vi "2_1_Face_Detection_Eval(CPU,GPU).vi"() -> ()   [LabVIEW 2020]
doc: "This example demonstrates the usage of the \"DeepLTK FPGA Addon\" for deploying a Face Detection model on a PXI-FPGA board, utilizing an input image sourced from a file.\n\nMore Examples: https://github.com/ngenehub/deepltk_fpga_examples"
uses:
  <vilib>/Ngene/Deep Learning Toolkit/Toolkit/NN_Network/Controls/NN_Device.ctl
  <vilib>/Ngene/Deep Learning Toolkit/Toolkit/NN_Network/Controls/NN_Save_Before_Destroy_Options.ctl
  723d4076-311b-47b4-ac66-0871b538cff2.vi
  <vilib>/Ngene/Deep Learning Toolkit/Toolkit/NN_Data/subVIs/Dataset/NN_Variant_to_DVR/4D/NN_Data_Variant_to_DVR(4D_SGL).vi
  <vilib>/Ngene/Deep Learning Toolkit/Toolkit/NN_Data/subVIs/Get_Data_Vals/4D/NN_Data_Get_ValByRef(4D_SGL_idx).vi
  <vilib>/Ngene/Deep Learning Toolkit/Toolkit/NN_Network/API/NN_Set_Input/3D/NN_Set_Input(3D_SGL_idx).vi
  <vilib>/Ngene/Deep Learning Toolkit/Toolkit/NN_Train/Eval_Loss/NN_Eval_Test_Error_Loss/NN_Eval(In3D_OutBBox).vi
  <vilib>/Ngene/Deep Learning Toolkit/Toolkit/NN_Train/Eval_Loss/NN_Calc_Cofusion_Matrix/NN_Calc_Confusion_Matrix(In3D_OutBBox).vi
  <vilib>/Ngene/Deep Learning Toolkit/Toolkit/Deep_Learning_Toolkit_by_Ngene.lvlib
  <vilib>/ptbypt/NI_PtbyPt.lvlib
panel:
  out "Eval Time":dbl=0.10011647000010271 format="%#_2p"
  out "Loop time":dbl=0.10057269999997516 format="%#_2p"
  out "Confusion Matrix":string[][](table)=[["24", "10", "0.7059"], ["8", "0", "0.0000"], ["0.7500", "0.0000", ""]]
  out "Iterations":i32=13
  out "Dataset Size":i32=14
  in  "NN_Device":T1
  in  "Stop":bool
  in  "Dataset Path (Annotations)":path=path "D:/Ngene/GitHub/deepltk_fpga_examples/2_Face_Detection(PXI,sbRIO)/Dataset/Annotations"
  out "mAP@0.5":sgl=0.72716737
  out "mIOU":sgl=0.5610681
  in  "Display?":bool
  out "Display":T2(plugin-control)
  in  "Dataset Path (Images)":path=path "D:/Ngene/GitHub/deepltk_fpga_examples/2_Face_Detection(PXI,sbRIO)/Dataset/Images"
  in  "Confidence_Thresh":sgl=0.46
  in  "IOU_Thresh":sgl=0.4
  in  "Weight File Path":path=path "D:/Ngene/GitHub/deepltk_fpga_examples/2_Face_Detection(PXI,sbRIO)/Models/Face_Detection_Original/Face_Detection.bin"
  in  "Configuration File Path":path=path "D:/Ngene/GitHub/deepltk_fpga_examples/2_Face_Detection(PXI,sbRIO)/Models/Face_Detection_Original/Face_Detection.cfg"
  # "Overview: This VI is designed to evaluate (measure the accuracy of) a pretrained object detection model.\nRequirements: \n• DeepLTK - Deep Learning Toolkit for LabVIEW (https://www.ngene.co/deep-learning-toolkit-for-labview)\n• NI Vision Development Module\nInstructions:\n1.\tProvide the path to the dataset to be evaluated at Dataset. A sample is available in the \"Dataset\" folder. \n2.\tProvide the \"Network Configuration File Path\" and \"Weight File Path\" locted in \"Models\\Face_Detection_Original\" folder in the project.\n3. Use NN_Device to specify the device (CPU or GPU) for execution. GPU is applicable only for 64-bit LabVIEW.\n4.\tRun the VI.\n5.\tObserve measured accuracy at mIOU, mAP@0.5 and Confusion Matrix indicators."
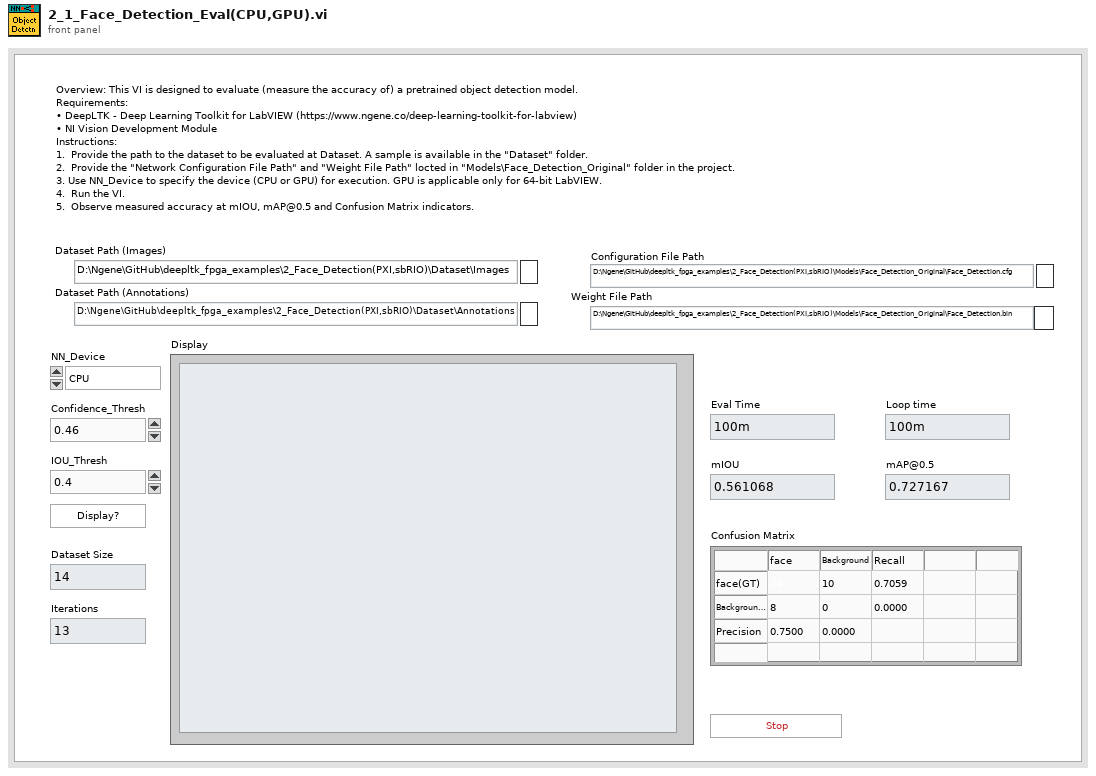
[diagram p1: front panel]
types:
  T1 = typedef "Deep_Learning_Toolkit_by_Ngene.lvlib/NN_Device.ctl" = enum16{"CPU", "GPU"}
  T2 = typedef "IMAQ Image.ctl" = refnum<image>
  T3 = typedef "Deep_Learning_Toolkit_by_Ngene.lvlib/NN_Save_Before_Destroy_Options.ctl" = cluster{"CFG?":bool, "Weights?":bool, "Render?":bool}
  T4 = typedef "Image Type" = u32
  T5 = typedef "Deep_Learning_Toolkit_by_Ngene.lvlib/NN_Config_Params.ctl" = cluster{"Name":string, "mBatch":i32, "NN_Train_Params":T6, "LR_Decay_Policy":T9, "Labels":string[], "Loss":T11}
  T6 = typedef "Deep_Learning_Toolkit_by_Ngene.lvlib/NN_Train_Params.ctl" = cluster{"Optimizer":T7, "Beta_1":sgl, "Beta_2":sgl, "Weight Decay(L1)":sgl, "Weight Decay(L2)":sgl, "Data_Sampling":T8}
  T7 = typedef "Deep_Learning_Toolkit_by_Ngene.lvlib/NN_Train_Optimizer.ctl" = enum16{"SGD", "Adam", "Adagrad", "Adadelta", "RMSProp", "Nesterov"}
  T8 = typedef "Deep_Learning_Toolkit_by_Ngene.lvlib/NN_Train_Data_Sampling.ctl" = enum16{"Random", "Sequential"}
  T9 = typedef "Deep_Learning_Toolkit_by_Ngene.lvlib/NN_LR_Policy_Cfg.ctl" = cluster{"Policy_Type":T10, "LR0":dbl, "k":sgl, "WarmUp_Policy":enum16{"Step", "Ramp"}, "WarmUp_Iter":i32, "WarmUp_Ratio":sgl}
  T10 = typedef "Deep_Learning_Toolkit_by_Ngene.lvlib/NN_LR_Policy_Type.ctl" = enum16{"Manual", "Step", "Exp", "1/t"}
  T11 = typedef "Deep_Learning_Toolkit_by_Ngene.lvlib/NN_Loss_Config_Params.ctl" = cluster{"Loss_Type":T12, "Loss_Conf_Params":variant}
  T12 = typedef "Deep_Learning_Toolkit_by_Ngene.lvlib/NN_Loss_Type.ctl" = enum16{"None", "MSE", "CrossEntropy", "YOLO_v2", "YOLO_v4"}
  T13 = typedef "Deep_Learning_Toolkit_by_Ngene.lvlib/NN_Layer_Config_Params.ctl" = cluster{"Layer_Type":T14, "Layer_Conf_Params":variant, "Input Layers":string[]}
  T14 = typedef "Deep_Learning_Toolkit_by_Ngene.lvlib/NN_Layer_Type.ctl" = enum16{"Input1D", "Input3D", "Conv1D", "Conv2D", "Conv2D_Adv", "MaxPool", "AvgPool", "UpSample", "DropOut3D", "ShortCut", "Concat", "SoftMax3D", "FC", "DropOut", "Softmax", "Flatten", "YOLO_v2", "YOLO_v4", "Activation", "BatchNormalization", "Unsupported"}
  T15 = typedef "Deep_Learning_Toolkit_by_Ngene.lvlib/NN.ctl" = cluster{"Name":string, "No of Layers":i32, "mBatch":i32, "Layers":T16[], "Dimty":T17, "Dims_In":T18, "Dims_Out":T18, "Working_Dir":path, "Train?":bool, "Train_Params":T6, "LR_Update_Policy":T9, "Session Data":T19, "Ground_truth":T20, "NNg_hdls":T21, "NN_Device":T1, "GPU Id":i32, "Labels":string[], "Receptive Field":T22[], "Loss_Type":T12, "Loss_Cfg_Prms":variant, "NNG_WS":T23}
  T16 = typedef "Deep_Learning_Toolkit_by_Ngene.lvlib/NN_Layer_ref.ctl" = refnum<data-value>
  T17 = typedef "Deep_Learning_Toolkit_by_Ngene.lvlib/NN_In_Out_Dim-ty.ctl" = enum8{"In1D_Out1D", "In3D_Out1D", "In3D_Out3D", "In3D_OutBBox"}
  T18 = typedef "Deep_Learning_Toolkit_by_Ngene.lvlib/NN_Dims(C,H,W).ctl" = cluster{"C":i32, "H":i32, "W":i32}
  T19 = typedef "Deep_Learning_Toolkit_by_Ngene.lvlib/NN_Train_Session_Data.ctl" = cluster{"Epochs":sgl, "Tot_Iter":i32, "LR":sgl, "LR_iter":i32}
  T20 = typedef "Deep_Learning_Toolkit_by_Ngene.lvlib/NN_Ground_truth.ctl" = cluster{"Y":variant}
  T21 = typedef "Deep_Learning_Toolkit_by_Ngene.lvlib/nng_cuda_handles.ctl" = cluster{"cudnn":u64, "cublas":u64, "stream":u64, "curand":u64}
  T22 = typedef "Deep_Learning_Toolkit_by_Ngene.lvlib/NN_Dims(V,H).ctl" = cluster{"V":i32, "H":i32}
  T23 = typedef "Deep_Learning_Toolkit_by_Ngene.lvlib/NNG_WS.ctl" = cluster{"NNG_WS_Mem":T24, "Max_WS_Size":i64}
  T24 = typedef "Deep_Learning_Toolkit_by_Ngene.lvlib/NNg_WS_Mem_DVR.ctl" = refnum<data-value>
  T25 = typedef "Deep_Learning_Toolkit_by_Ngene.lvlib/NN_DataSets_All(In3D_OutBBox).ctl" = cluster{"Train":T26, "Validation":T26, "Test":T26}
  T26 = typedef "Deep_Learning_Toolkit_by_Ngene.lvlib/NN_DataSet(In3D_OutBBox).ctl" = cluster{"Inputs Ref.":variant, "Dataset_Size":i32, "Dims_In":T18, "Outputs Refs":T27, "No of Classes ":i32, "Labels":string[], "File Paths":path[]}
  T27 = typedef "Deep_Learning_Toolkit_by_Ngene.lvlib/NN_Data_ref(1D_BBox).ctl" = refnum<data-value>
  T28 = typedef "Deep_Learning_Toolkit_by_Ngene.lvlib/NN_Data_ref(4D_SGL).ctl" = refnum<data-value>
  T29 = typedef "Deep_Learning_Toolkit_by_Ngene.lvlib/NN_Layer.ctl" = cluster{"Name":string, "Layer_Data":variant, "Layer_Type":T14, "Dims_In":T18, "Layers_In":variant, "Dims_Out":T18, "Layers_Out":variant, "Metrics":T30, "GPU_Data":variant, "mBatch":i32, "NN_Device":T1, "NNg_hdls":T21, "Train?":bool, "Dimty":T31, "RecptField":T32}
  T30 = typedef "Deep_Learning_Toolkit_by_Ngene.lvlib/NN_Layer_Metrics.ctl" = cluster{"Data":dbl, "Params":dbl, "Ops":dbl}
  T31 = typedef "Deep_Learning_Toolkit_by_Ngene.lvlib/NN_Layer_Dimty.ctl" = enum16{"1D", "3D"}
  T32 = typedef "Deep_Learning_Toolkit_by_Ngene.lvlib/NN_Layer_RF_State.ctl" = cluster{"Dims":T22, "J":T22}
  T33 = typedef "Deep_Learning_Toolkit_by_Ngene.lvlib/NN_BBox_Detection.ctl" = cluster{"Class":i32, "Conf Level":sgl, "BBox":T34}
  T34 = typedef "Deep_Learning_Toolkit_by_Ngene.lvlib/NN_BBox.ctl" = cluster{"x":sgl, "y":sgl, "w":sgl, "h":sgl}
  T35 = typedef "Deep_Learning_Toolkit_by_Ngene.lvlib/NN_Eval_Params(in3D_OutBBox).ctl" = cluster{"Precision@Max_Avg_F1_Score":sgl, "Recall@Max_Avg_F1_Score":sgl, "argmax_avgF1_Score(Conf)":sgl, "Max_Avg_F1_Score":sgl, "Max_F1_Score_Per_Class":sgl[], "F1_Score_Per_Class":sgl[][], "Avg_F1,P,R Curves":cluster{"Conf":sgl[], "F1|P|R":sgl[]}[], "mIOU":sgl, "APs@0.5":sgl[], "PR_Curves@0.5":T36, "IOUs":sgl[], "mAP@0.75":sgl, "mAP@0.5-0.95":sgl, "mAP@0.5":sgl, "Mean_PR_Curve":T37}
  T36 = typedef "Deep_Learning_Toolkit_by_Ngene.lvlib/NN_PR_Curves.ctl" = T37[]
  T37 = typedef "Deep_Learning_Toolkit_by_Ngene.lvlib/NN_PR.ctl" = cluster{"Recall":sgl[], "Precision":sgl[]}
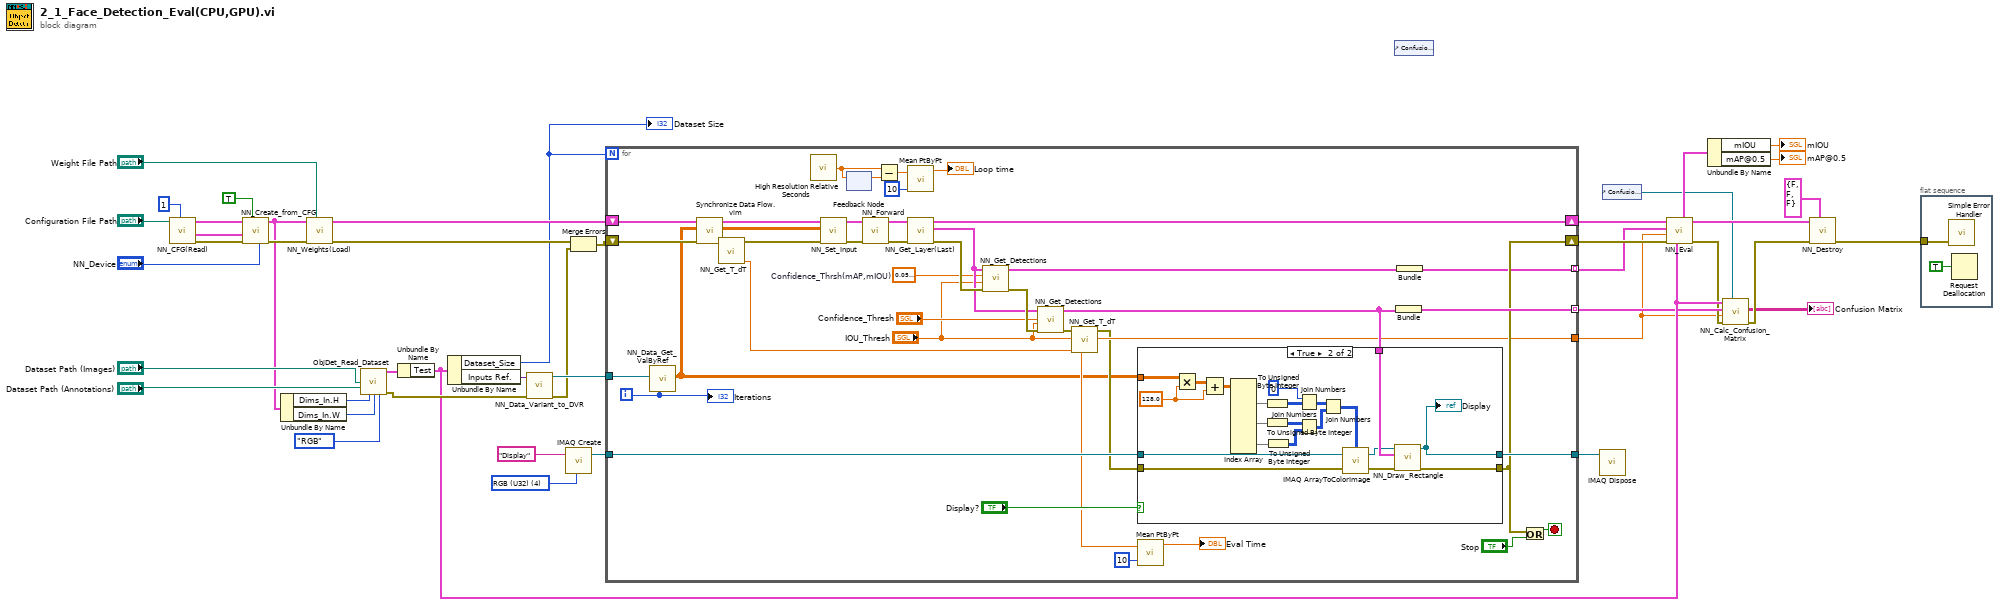
[diagram p0: block diagram]
diagram:
  w42 = T4 4 items=["Grayscale (U8)", "Grayscale (I16)", "Grayscale (SGL)", "Complex (CSG)", "RGB (U32)", "HSL (U32)", "RGB (U64)", "Grayscale (U16)"] ("Image Type")
  n1 = call <vilib>:"NN_CFG(Read).vi"("mBatch"=1, "CFG file path"="Configuration File Path") -> ("error out"=w25:errorcluster, "Net_Cfg"=w23:T5, "Layer_Cfg"=w20:T13[])  [unwired: 7 in]
  n2 = call <vilib>:"NN_Create_from_CFG.vi"("NN_Device"="NN_Device", "Train? (false)"=TRUE, "error in (no error)"=w25, "Net_Cfg"=w23, "Layer_Cfg"=w20) -> ("error out"=w24:errorcluster, "NN out"=w4:T15)  [unwired: 5 in]
  n3 = Unbundle By Name(w4) -> ("Dims_In.H"=w3:i32, "Dims_In.W"=w2:i32)
  n4 = call <vilib>:"NN_Weights(Load).vi"("Weight File Path"="Weight File Path", "error in (no error)"=w24, "NN in"=w4) -> ("error out"=w18:errorcluster, "NN out"=w19:T15)  [unwired: 7 in]
  n5 = call "ObjDet_Read_Dataset.vi"("Image Path(Test)"="Dataset Path (Images)", "Anno Path(Test)"="Dataset Path (Annotations)", "Img Height"=w3, "Img Width"=w2, "Img Type"=enum16{"Grayscale", "RGB"}."RGB") -> ("Dataset"=w40:T25, "error out"=w29:errorcluster)  [unwired: 7 in, 2 out]
  n6 = Unbundle By Name(w40) -> ("Test"=w12:T26)
  n7 = Unbundle By Name(w12) -> ("Dataset_Size"=w13:i32, "Inputs Ref."=w39:variant)
  "Dataset Size" <- w13
  n8 = call-poly <vilib>:"NN_Data_Variant_to_DVR.vi"("error in (no error)"=w29, "Inputs Ref."=w39) -> ("error out"=w27:errorcluster, "DVR(4D_SGL)"=w38:T28)  [unwired: 8 in]
  n9 = call "IMAQ Create"("Image Name"="Display", "Image Type"=w42) -> ("New Image"=w43:T2)  [unwired: 3 in, 1 out]
  n10 = Merge Errors(w18, w27) -> (w28:errorcluster)
  n11 = for {
    N: w13 -> [_]
    shift-right: [w69] -> w36
    shift-left: w19 -> [w51]
    tunnel: w43 -> [w80]
    shift-right: [w74] -> w32
    shift-left: w28 -> [w50]
    tunnel: w38 -> [w82]
    tunnel: [w79] -> w11 mode=indexing
    tunnel: [w78] -> w37
    tunnel: ["IOU_Thresh"] -> w7
    tunnel: [w61] -> w1 mode=indexing
    i -> [w68]
    stop <- w73 stop-if-true
    w58 = sgl 0.05  # Confidence_Thrsh(mAP,mIOU)
    # "Inference Loop"
    n12 = call-poly <vilib>:"NN_Data_Get_ValByRef.vi"("index (vol)"=w68, "DVR(4D_SGL)"=w82) -> ("Value(3D_SGL)"=w48:sgl[][][])  [unwired: 6 in, 1 out]
    n13 = call "Synchronize Data Flow.vim"("input 4"=w50, "input 2"=w48, "input 1"=w51) -> ("output 4"=w49:errorcluster, "output 2"=w47:sgl[][][], "output 1"=w46:T15)  [unwired: 1 in, 1 out]
    n14 = call <vilib>:"NN_Get_T_dT.vi"("error in (no error)"=w49) -> ("T_out"=w54:dbl, "error out"=w56:errorcluster)  [unwired: 6 in, 1 out]
    n15 = call <vilib>:"High Resolution Relative Seconds.vi"() -> ("relative seconds"=w76:dbl)
    n16 = call-poly <vilib>:"NN_Set_Input.vi"("error in (no error)"=w56, "Data_In(3D_SGL)"=w47, "NN in"=w46) -> ("error out"=w84:errorcluster, "NN out"=w85:T15)  [unwired: 7 in]
    n17 = feedback #1() -> (w77:dbl)  [unwired: 1 in]
    n18 = feedback-in #1(w76) -> ()
    n19 = call <vilib>:"NN_Forward.vi"("error in (no error)"=w84, "NN in"=w85) -> ("error out"=w83:errorcluster, "NN out"=w70:T15)  [unwired: 6 in, 2 out]
    n20 = Subtract(x=w76, y=w77) -> (x-y=w75:dbl)
    n21 = call <vilib>:"Mean PtByPt.vi"("x"=w75, "sample length"=10) -> ("mean"=→"Loop time":dbl)  [unwired: 2 in, 1 out]
    n22 = call <vilib>:"NN_Get_Layer(Last).vi"("error in (no error)"=w83, "NN in"=w70) -> ("error out"=w71:errorcluster, "Last_Layer"=w65:T29, "NN out"=w69:T15)  [unwired: 6 in, 1 out]
    n23 = call <vilib>:"NN_Get_Detections.vi"("error in"=w71, "IOU_Thrsh"="IOU_Thresh", "Confidence_Thrsh"=w58, "YOLO_Layer"=w65) -> ("error out"=w66:errorcluster, "Detections"=w62:T33[])  [unwired: 6 in]
    n24 = call <vilib>:"NN_Get_Detections.vi"("error in"=w66, "IOU_Thrsh"="IOU_Thresh", "Confidence_Thrsh"="Confidence_Thresh", "YOLO_Layer"=w65) -> ("error out"=w63:errorcluster, "Detections"=w64:T33[])  [unwired: 6 in]
    n25 = call <vilib>:"NN_Get_T_dT.vi"("T_in"=w54, "error in (no error)"=w63) -> ("error out"=w55:errorcluster, "dT"=w53:dbl)  [unwired: 5 in, 1 out]
    n26 = case shown="True" "Display?" {
      tunnel: w55 -> [w87 w108]
      tunnel: w80 -> [w86 w107]
      tunnel: w64 -> [_ w97]
      tunnel: [w87 w94] -> w74
      tunnel: w48 -> [_ w93]
      tunnel: [w86 w90] -> w78
      frame False {
      }
      frame True {
        w88 = sgl 128.0 ("x")
        n27 = Multiply(x=w93, y=w88) -> (x*y=w89:sgl[][][])
        n28 = Add(x=w89, y=w88) -> (x+y=w95:sgl[][][])
        n29 = Index Array(array=w95) -> (element #1=w106:sgl[][], element #2=w103:sgl[][], element #3=w101:sgl[][])  [unwired: 9 in]
        n30 = To Unsigned Byte Integer(number=w106) -> (unsigned 8bit integer=w105:u8[][])
        n31 = To Unsigned Byte Integer(number=w103) -> (unsigned 8bit integer=w102:u8[][])
        n32 = To Unsigned Byte Integer(number=w101) -> (unsigned 8bit integer=w100:u8[][])
        n33 = Join Numbers(hi=u8 0, lo=w105) -> ((hi.lo)=w104:u16[][])
        n34 = Join Numbers(hi=w102, lo=w100) -> ((hi.lo)=w99:u16[][])
        n35 = Join Numbers(hi=w104, lo=w99) -> ((hi.lo)=w92:u32[][])
        n36 = call "IMAQ ArrayToColorImage"("Image Pixels (U32)"=w92, "Image"=w107, "error in (no error)"=w108) -> ("Image Out"=w96:T2, "error out"=w91:errorcluster)  [unwired: 2 in]
        n37 = call "NN_Draw_Rectangle.vi"("error in (no error)"=w91, "Draw_Boxes"=w97, "Image_in"=w96) -> ("error out"=w94:errorcluster, "Image_out"=w90:T2)  [unwired: 6 in, 1 out]
        "Display" <- w90
      }
    }
    n38 = call <vilib>:"Mean PtByPt.vi"("x"=w53, "sample length"=10) -> ("mean"=→"Eval Time":dbl)  [unwired: 2 in, 1 out]
    n39 = Bundle("Detections"=w64) -> (w79:cluster{"Detections":T33[]})  [unwired: 1 in]
    n40 = Bundle("Detections"=w62) -> (w61:cluster{"Detections":T33[]})  [unwired: 1 in]
    n41 = Or(x=w74, y="Stop") -> (x .or. y?=w73:bool)
    "Iterations" <- w68
  }
  n42 = control-ref of="Confusion Matrix"() -> ()  [unwired: 1 out]
  n43 = call "IMAQ Dispose"("Image"=w37) -> ()  [unwired: 5 in, 1 out]
  n44 = control-ref of="Confusion Matrix"() -> (w5:refnum<vi>)
  n45 = call-poly <vilib>:"NN_Eval.vi"("Dataset"=w12, "error in"=w32, "IOU_Conf_Thrsh(0.5)"=w7, "Detections(in Dataset)"=w1, "NN in"=w36) -> ("error out"=w10:errorcluster, "NN out"=w15:T15, "NN_Eval_Params"=w35:T35)  [unwired: 4 in]
  n46 = Unbundle By Name(w35) -> ("mIOU"=→"mIOU":sgl, "mAP@0.5"=→"mAP@0.5":sgl)
  n47 = call-poly <vilib>:"NN_Calc_Confusion_Matrix.vi"("Confusion Matrix (Table) ref."=w5, "error in (no error)"=w10, "TP_IOU_Thrsh(0.5)"=w7, "Predictions"=w11, "Dataset"=w12) -> ("error out"=w9:errorcluster, "Confusion Matrix (Table)"=→"Confusion Matrix":string[][])  [unwired: 3 in, 2 out]
  n48 = call <vilib>:"NN_Destroy.vi"("Save (T, T, T)"=T3 {"CFG?"=FALSE, "Weights?"=FALSE, "Render?"=FALSE}, "error in (no error)"=w9, "NN in"=w15) -> ("error out"=w41:errorcluster)  [unwired: 7 in, 1 out]
  n49 = flat-sequence {
    tunnel: w41 -> [w109]
    frame #0 {
      n50 = call <vilib>:"Simple Error Handler.vi"("error in (no error)"=w109) -> ()  [unwired: 4 in, 5 out]
      n51 = Request Deallocation(TRUE ("flag")) -> ()
    }
  }
